vi "check interlock channels.vi"(7 "RT Queues in":T9, 9 "scaledData":dbl[][](array[numeric]), 11 "Data in":T2={"Parameters"={"FPGA Ref"=refnum, "data stream"={"data writer name"="error writer", "NS write buffer size"=16, "NS Buffer length"=0}, "FIFO Depth"=0, "Channel controls"={"FIFO channel count"=0, "active indices"=[], "active channels"=0, "channelScaling"=[], "scanivalveCount"=0, "channels"=[]}, "safetyChannels"={"oilP"=0, "airP"=0, "water"=0, "channelLimits"=[]}, "speedChannel"=0, "maxSpeedLimit"=0.0, "Torque"={"fixedOffset"=0.0, "filter"=FALSE, "fallingEdge"=FALSE, "swapEncoders"=FALSE}}, "Variables"={"Intermediary buffer"=[], "buffer position"=0, "write loop counter"=0, "NS write trigger"=0, "NS Connection status"=FALSE, "waiting for NS"=FALSE, "labAmbient"={"pressure"=0.0, "temperature"=0.0}, "scanivalvePorts"=[], "scanivalvePressures"=[], "data stream"="", "activeChannelLimitIndex"=[], "runningSpeedLimit"=0.0, "speedChannelIndex"=0, "Interlocks"={"gearboxOil"=FALSE, "bearingOil"=FALSE, "gearboxAir"=FALSE}, "interlockChannels"={"gearboxOil"=0, "bearingOil"=0, "air"=0}, "limitStates"=[]}}) -> (3 "Data out":T2={"Parameters"={"FPGA Ref"=refnum, "data stream"={"data writer name"="error writer", "NS write buffer size"=16, "NS Buffer length"=0}, "FIFO Depth"=0, "Channel controls"={"FIFO channel count"=0, "active indices"=[], "active channels"=0, "channelScaling"=[], "scanivalveCount"=0, "channels"=[]}, "safetyChannels"={"oilP"=0, "airP"=0, "water"=0, "channelLimits"=[]}, "speedChannel"=0, "maxSpeedLimit"=0.0, "Torque"={"fixedOffset"=0.0, "filter"=FALSE, "fallingEdge"=FALSE, "swapEncoders"=FALSE}}, "Variables"={"Intermediary buffer"=[], "buffer position"=0, "write loop counter"=0, "NS write trigger"=0, "NS Connection status"=FALSE, "waiting for NS"=FALSE, "labAmbient"={"pressure"=0.0, "temperature"=0.0}, "scanivalvePorts"=[], "scanivalvePressures"=[], "data stream"="", "activeChannelLimitIndex"=[], "runningSpeedLimit"=0.0, "speedChannelIndex"=0, "Interlocks"={"gearboxOil"=FALSE, "bearingOil"=FALSE, "gearboxAir"=FALSE}, "interlockChannels"={"gearboxOil"=0, "bearingOil"=0, "air"=0}, "limitStates"=[]}})   [LabVIEW 2018]
uses:
  Type Defs/Queues cluster.ctl
  ICL-LabVIEW_General/Message Scheduler/message scheduler.lvclass
  Type Defs/Data processing loop data.ctl
  Type Defs/FPGA reference.ctl
  PC/type defs/channelControl.ctl
  Type Defs/channelScalingTypes.ctl
  Type Defs/scalingMethods.ctl
  ICL-LabVIEW_General/data channels/parent class/Data Channel.lvclass
  PC/type defs/channelLimitControl.ctl
  PC/type defs/limitActions.ctl
  Queue VIs/En-queue RT message element.vi
panel:
  out "Interlocks":T1
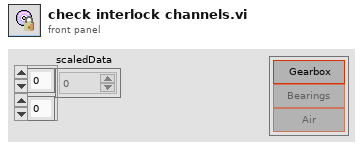
[diagram p1: front panel]
types:
  T1 = cluster{"gearboxOil":bool, "bearingOil":bool, "gearboxAir":bool}
  T2 = typedef "Data processing loop data.ctl" = cluster{"Parameters":cluster{"FPGA Ref":T3, "data stream":cluster{"data writer name":string, "NS write buffer size":i32, "NS Buffer length":u32}, "FIFO Depth":u32, "Channel controls":cluster{"FIFO channel count":i32, "active indices":i16[], "active channels":i32, "channelScaling":T4[], "scanivalveCount":i32, "channels":refnum<class "Data Channel.lvclass">[]}, "safetyChannels":cluster{"oilP":u16, "airP":u16, "water":u16, "channelLimits":T7[]}, "speedChannel":i32, "maxSpeedLimit":dbl, "Torque":cluster{"fixedOffset":dbl, "filter":bool, "fallingEdge":bool, "swapEncoders":bool}}, "Variables":cluster{"Intermediary buffer":dbl[][], "buffer position":u32, "write loop counter":u16, "NS write trigger":u32, "NS Connection status":bool, "waiting for NS":bool, "labAmbient":cluster{"pressure":dbl, "temperature":dbl}, "scanivalvePorts":u16[], "scanivalvePressures":dbl[], "data stream":refnum<k21>, "activeChannelLimitIndex":u16[], "runningSpeedLimit":dbl, "speedChannelIndex":i32, "Interlocks":cluster{"gearboxOil":bool, "bearingOil":bool, "gearboxAir":bool}, "interlockChannels":cluster{"gearboxOil":i32, "bearingOil":i32, "air":i32}, "limitStates":cluster{"warn":bool, "alarm":bool}[]}}
  T3 = typedef "FPGA reference.ctl" = refnum<k20>
  T4 = typedef "channelControl.ctl" = cluster{"index":u16, "active":bool, "channelType":T5, "module":u16, "terminal":u16, "channelName":string, "scalingMethod":T6, "scalingParameters":dbl[], "scaledUnits":string, "tempOffset":dbl}
  T5 = typedef "channelScalingTypes.ctl" = enum16{"calculation", "measurement", "scanivalve", "output", "digital"}
  T6 = typedef "scalingMethods.ctl" = enum16{"none", "linear", "thermocouple", "polynomial", "encoder", "RTD"}
  T7 = typedef "channelLimitControl.ctl" = cluster{"channelID":u16, "Enabled":bool, "warnValue":dbl, "limitValue":dbl, "Invert":bool, "limitAction":T8}
  T8 = typedef "limitActions.ctl" = enum16{"stop", "shutdown", "ignore"}
  T9 = typedef "Queues cluster.ctl" = cluster{"RT Message":refnum<queue>, "RT Comms":refnum<queue>, "RT Data":refnum<queue>, "RT FIFO":refnum<queue>, "message scheduler":refnum<class "message scheduler.lvclass">}
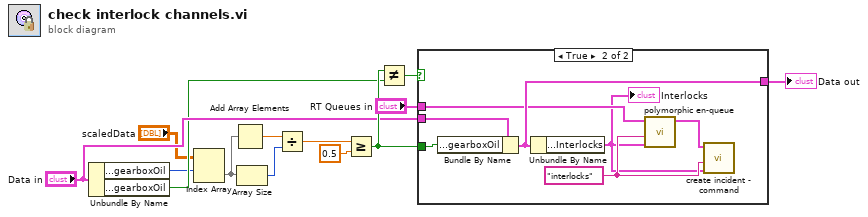
[diagram p0: block diagram]
diagram:
  n1 = Unbundle By Name("Data in") -> ("Variables.interlockChannels.gearboxOil"=w5:i32, "Variables.Interlocks.gearboxOil"=w8:bool)
  n2 = Index Array(array="scaledData", index (row)=w5) -> (element=w6:dbl[])  [unwired: 1 in]
  n3 = Add Array Elements(numeric array=w6) -> (sum=w1:dbl)
  n4 = Array Size(array=w6) -> (size(s)=w2:i32)
  n5 = Divide(x=w1, y=w2) -> (x/y=w3:dbl)
  n6 = Greater Or Equal?(x=w3, y=0.5) -> (x >= y?=w11:bool)
  n7 = Not Equal?(x=w11, y=w8) -> (x != y?=w9:bool)
  n8 = case shown="True" w9 {
    tunnel: "Data in" -> [w14 w21]
    tunnel: [w14 w19] -> w12
    tunnel: w11 -> [_ w20]
    tunnel: "RT Queues in" -> [_ w18]
    frame False {
    }
    frame True {
      w16 = "interlocks" ("Message")
      n9 = Bundle By Name(cluster=w21, "Variables.Interlocks.gearboxOil"=w20) -> (w19:T2)
      n10 = Unbundle By Name(w19) -> ("Variables.Interlocks"=w15:T1)
      "Interlocks" <- w15
      n11 = call-poly "polymorphic en-queue.vi"("Data"=w15, "Message"=w16, "RT Queues"=w18) -> ("RT Queues out"=w17:T9)  [unwired: 8 in]
      n12 = call "create incident - command.vi"("data"=w15, "command"=w16, "RT Queues"=w17) -> ()  [unwired: 9 in]
    }
  }
  "Data out" <- w12
